vi "alter database password.vi"(8 "错误输入（无错误）":errorcluster, 9 "NewPWd":string, 10 "OpenPwd":string, 11 "路径":path) -> (0 "错误输出":errorcluster)   [LabVIEW 2016, in "Access Lib.lvlib"]
uses:
  Access Lib.lvlib
  <vilib>/addons/database/Connection.llb/DB Tools Open Connec (String).vi
  <vilib>/addons/database/Connection.llb/Conn Execute.vi
  <vilib>/addons/database/Recordset.llb/Rec Destroy - Connection.vi
  <vilib>/addons/database/NI_Database_API.lvlib
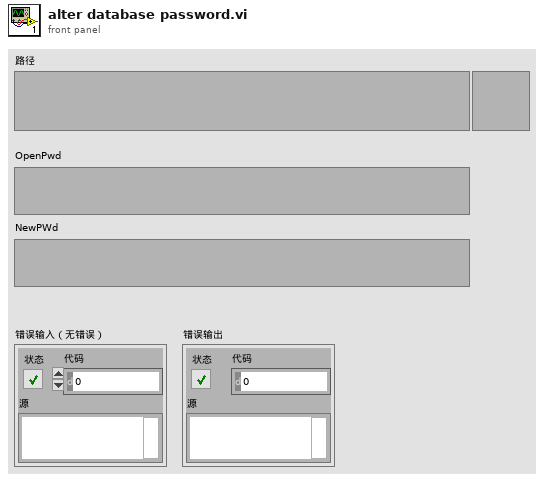
[diagram p1: front panel]
types:
  T1 = typedef "NI_Database_API.lvlib/Conn ObjectReference.ctl" = refnum<k1>
  T2 = typedef "NI_Database_API.lvlib/Rec ObjectReference.ctl" = refnum<k1>
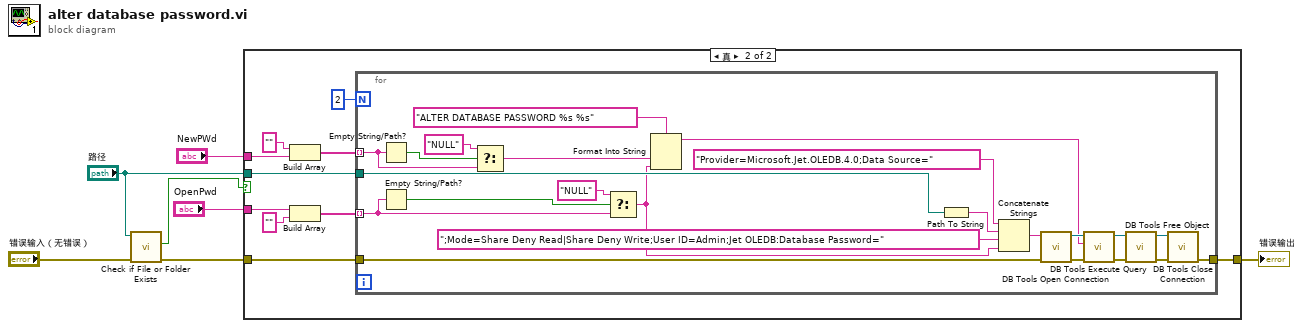
[diagram p0: block diagram]
diagram:
  n1 = call <vilib>:"Check if File or Folder Exists.vi"("error in (no error)"="错误输入（无错误）", "path"="路径") -> ("error out"=w3:errorcluster, "file or folder exists?"=w5:bool)  [unwired: 7 in, 1 out]
  n2 = case shown="真" w5 {
    tunnel: "OpenPwd" -> [_ w14]
    tunnel: "路径" -> [_ w18]
    tunnel: w3 -> [w8 w16]
    tunnel: [w8 w17] -> w2
    tunnel: "NewPWd" -> [_ w10]
    frame False {
    }
    frame True {
      n3 = Build Array("", w10) -> (w9:string[])
      n4 = Build Array(w14, "") -> (w12:string[])
      n5 = for {
        N: 2 -> [_]
        tunnel: w18 -> [w38]
        tunnel: w9 -> [w24] mode=indexing
        tunnel: w12 -> [w21] mode=indexing
        tunnel: w16 -> [w29]
        tunnel: [w30] -> w17
        n6 = Empty String/Path?(string/path=w24) -> (empty?=w26:bool)
        n7 = Empty String/Path?(string/path=w21) -> (empty?=w22:bool)
        n8 = Select(t="NULL", s=w26, f=w24) -> (s? t:f=w20:string)
        n9 = Select(t="NULL", s=w22, f=w21) -> (s? t:f=w19:string)
        n10 = Format Into String(format string="ALTER DATABASE PASSWORD %s %s" ("格式字符串"), w20, w19) -> (resulting string=w27:string)  [unwired: 2 in, 1 out]
        n11 = Path To String(path=w38) -> (string=w41:string)
        n12 = Concatenate Strings("Provider=Microsoft.Jet.OLEDB.4.0;Data Source=" ("ConnectString"), w41, ";Mode=Share Deny Read|Share Deny Write;User ID=Admin;Jet OLEDB:Database Password=" ("字符串"), w19) -> (w37:string)
        n13 = call-poly <vilib>:"DB Tools Open Connection.vi"("error in (no error)"=w29, "connection information"=w37) -> ("error out"=w35:errorcluster, "connection reference"=w36:T1)  [unwired: 6 in]
        n14 = call-poly <vilib>:"DB Tools Execute Query.vi"("error in (no error)"=w35, "SQL query"=w27, "connection reference"=w36) -> ("error out"=w33:errorcluster, "recordset reference"=w34:T2)  [unwired: 5 in]
        n15 = call-poly <vilib>:"DB Tools Free Object.vi"("error in (no error)"=w33, "recordset reference"=w34) -> ("error out"=w31:errorcluster, "connection reference"=w32:T1)  [unwired: 8 in]
        n16 = call <vilib>:"DB Tools Close Connection.vi"("error in (no error)"=w31, "connection reference"=w32) -> ("error out"=w30:errorcluster)  [unwired: 5 in]
      }
    }
  }
  "错误输出" <- w2
